vi "Dequeue Message.vi"(6 "timeout in ms (-1)":i32=-1, 8 "error in (no error)":errorcluster, 11 "Message Queue":refnum<queue>) -> (0 "error out":errorcluster, 1 "Message Data":variant, 2 "Message":string, 3 "dup Message Queue":refnum<queue>, 4 "timed out?":bool)   [LabVIEW 2023, in "Front Panel Message Queue.lvlib"]
uses:
  Front Panel Message Queue.lvlib
  Message Cluster.ctl
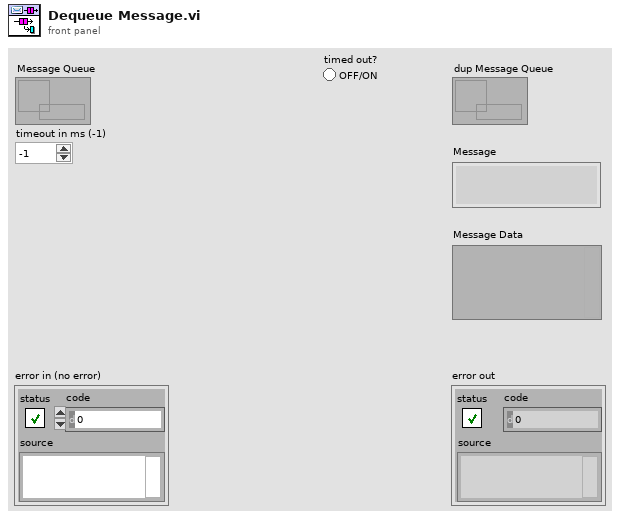
[diagram p1: front panel]
types:
  T1 = typedef "Front Panel Message Queue.lvlib/Message Cluster.ctl" = cluster{"Message":string, "Message Data":variant}
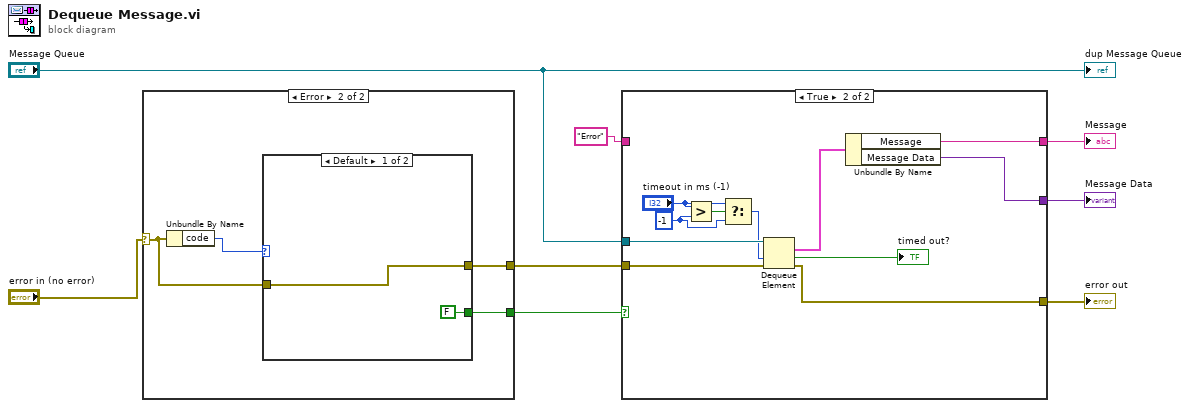
[diagram p0: block diagram]
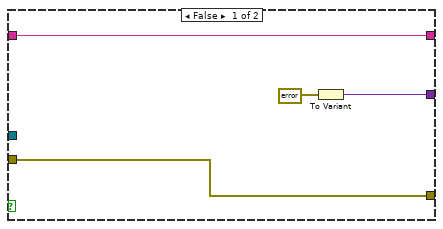
[diagram p2: hidden frame]
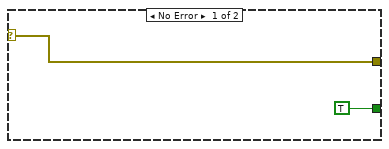
[diagram p3: hidden frame]
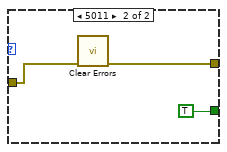
[diagram p4: hidden frame]
diagram:
  n1 = case shown="Error" "error in (no error)" {
    selector: "error in (no error)" -> [w10 w12]
    tunnel: [w10 w11] -> w3
    tunnel: [TRUE w13] -> w2
    frame No Error {
    }
    frame Error {
      n2 = Unbundle By Name(w12) -> ("code"=w14:i32)
      n3 = case shown="Default" w14 {
        tunnel: [FALSE TRUE] -> w13
        tunnel: w12 -> [w15 w18]
        tunnel: [w15 w17] -> w11
        frame Default {
        }
        frame 5011 {
          n4 = call <vilib>:"Clear Errors.vi"("error in (no error)"=w18) -> ("error out"=w17:errorcluster)  [unwired: 5 in, 1 out]
        }
      }
    }
  }
  n5 = case shown="True" w2 {
    tunnel: "Message Queue" -> [_ w34]
    tunnel: [w23 w33] -> w7
    tunnel: [w21 w32] -> w6
    tunnel: [w20 w30] -> w5
    tunnel: w3 -> [w20 w29]
    tunnel: "Error" -> [w23 _]
    frame False {
      n6 = To Variant(anything=errorcluster {"status"=FALSE, "code"=0, "source"=""} ("error constant")) -> (Variant=w21:variant)
    }
    frame True {
      w25 = -1
      n7 = Greater?(x="timeout in ms (-1)", y=w25) -> (0:w26:bool)
      n8 = Select(t="timeout in ms (-1)", s=w26, f=w25) -> (s? t:f=w24:i32)
      n9 = Dequeue Element(queue=w34, timeout in ms (-1)=w24, error in (no error)=w29) -> (element=w31:T1, timed out?=→"timed out?":bool, error out=w30:errorcluster)  [unwired: 1 out]
      n10 = Unbundle By Name(w31) -> ("Message"=w33:string, "Message Data"=w32:variant)
    }
  }
  "error out" <- w5
  "Message" <- w7
  "Message Data" <- w6
  "dup Message Queue" <- "Message Queue"
